vi "GetControllerData.vi"(8 "error in (no error)":errorcluster, 11 "device ID":refnum<k1>) -> (0 "error out":errorcluster, 1 "Buttons":bool[](array[boolean]), 2 "Axes":dbl[](array[numeric]), 3 "device ID 2":refnum<k1>, 4 "Directional":i32[](array[numeric]))   [LabVIEW 2014]
uses:
  <vilib>/Utility/inputDevices.llb/joystickAcquire.vi
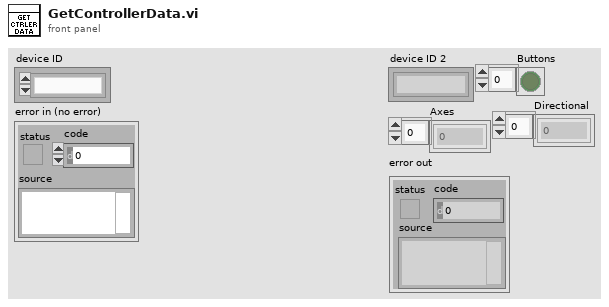
[diagram p1: front panel]
types:
  T1 = cluster{"X axis":i32, "Y axis":i32, "Z axis":i32, "X axis rotation":i32, "Y axis rotation":i32, "Z axis rotation":i32, "U axis":i32, "V axis":i32}
  T2 = cluster{"button 1":bool, "button 2":bool, "button 3":bool, "button 4":bool, "button 5":bool, "button 6":bool, "button 7":bool, "button 8":bool, "button 9":bool, "button 10":bool, "button 11":bool, "button 12":bool, "button 13":bool, "button 14":bool, "button 15":bool, "button 16":bool, "button 17":bool, "button 18":bool, "button 19":bool, "button 20":bool, "button 21":bool, "button 22":bool, "button 23":bool, "button 24":bool, "button 25":bool, "button 26":bool, "button 27":bool, "button 28":bool, "button 29":bool, "button 30":bool, "button 31":bool, "button 32":bool}
  T3 = cluster{"pov 1":i32, "pov 2":i32, "pov 3":i32, "pov 4":i32}
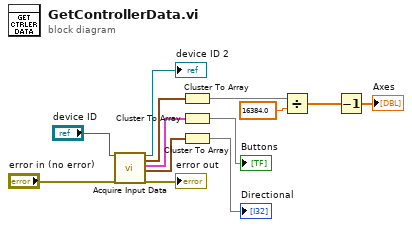
[diagram p0: block diagram]
diagram:
  n1 = call-poly <vilib>:"Acquire Input Data.vi"("device ID"="device ID", "error in (no error)"="error in (no error)") -> ("device ID"=→"device ID 2":refnum<k1>, "axis info"=w11:T1, "button info"=w10:T2, "direction info"=w9:T3, "error out"=→"error out":errorcluster)  [unwired: 13 in]
  n2 = Cluster To Array(cluster=w11) -> (array=w7:i32[])
  n3 = Cluster To Array(cluster=w10) -> (array=→"Buttons":bool[])
  n4 = Cluster To Array(cluster=w9) -> (array=→"Directional":i32[])
  n5 = Divide(x=w7, y=16384.0) -> (x/y=w6:dbl[])
  n6 = Decrement(x=w6) -> (x-1=→"Axes":dbl[])
